vi "GF_SetRecordLengthProperly.vi"(2 "error in (no error)":errorcluster, 3 "Num Samples":T1(ring), 4 "VISA resource name":refnum<visa-resource-name>) -> (0 "error out":errorcluster, 1 "VISA resource name out":refnum<visa-resource-name>)   [LabVIEW 2020]
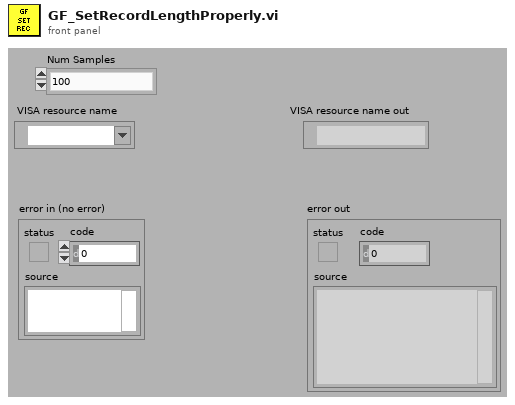
[diagram p1: front panel]
types:
  T1 = enum16{"100", "250", "500", "1000", "2000", "5000", "10000", "20000", "50000", "100000", "200000", "500000", "1000000", "2000000", "4000000", "8000000"}
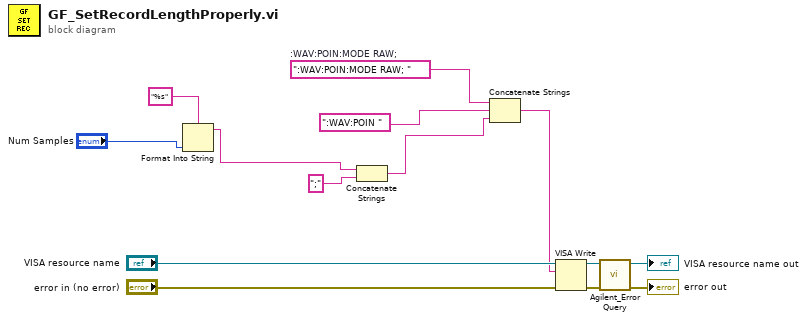
[diagram p0: block diagram]
diagram:
  w2 = ":WAV:POIN:MODE RAW; "  # :WAV:POIN:MODE RAW;
  n1 = Format Into String(format string="%s", "Num Samples") -> (resulting string=w1:string)  [unwired: 2 in, 1 out]
  n2 = Concatenate Strings(w1, ";" ("string")) -> (w12:string)
  n3 = Concatenate Strings(w2, ":WAV:POIN ", w12) -> (w3:string)
  n4 = VISA Write(VISA resource name="VISA resource name", write buffer=w3, error in (no error)="error in (no error)") -> (VISA resource name out=w5:refnum<visa-resource-name>, error out=w4:errorcluster)  [unwired: 1 out]
  n5 = call "Agilent_Error Query.vi"("error in (no error)"=w4, "VISA resource name"=w5) -> ("error out"=→"error out":errorcluster, "VISA resource name out"=→"VISA resource name out":refnum<visa-resource-name>)  [unwired: 6 in, 2 out]
